vi "Audio.Sound Recorder.vi"() -> ()   [LabVIEW 2018]
uses:
  <vilib>/sound2/lvsound2.llb/Sampling Mode.ctl
  <vilib>/Utility/sysdir.llb/System Directory Type.ctl
  <vilib>/sound2/lvsound2.llb/Sound Input Read (DBL).vi
panel:
  in  "Exit":bool
  out "Active":bool
  in  "Record":bool
  in  "Duration(s)":dbl=5.0 format="%#_13g"
  # "Sound Recorder"
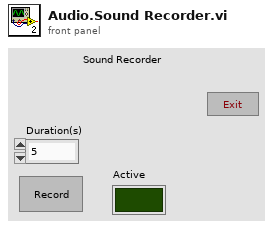
[diagram p1: front panel]
types:
  T1 = typedef "System Directory Type.ctl" = i32
  T2 = typedef "Sampling Mode.ctl" = i32
  T3 = typedef "Sound Input Task ID.ctl" = u32
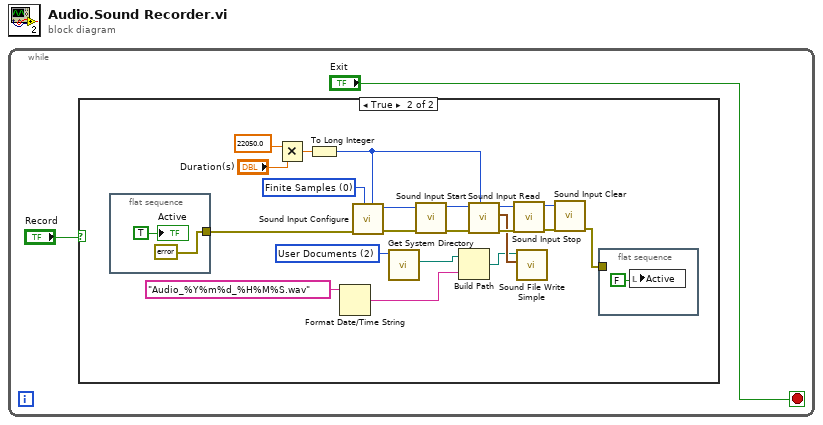
[diagram p0: block diagram]
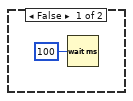
[diagram p2: hidden frame]
diagram:
  n1 = while {
    stop <- "Exit" stop-if-true
    n2 = case shown="True" "Record" {
      frame False {
        n3 = Wait (ms)(milliseconds to wait=u32 100) -> ()  [unwired: 1 out]
      }
      frame True {
        w8 = T1 2 items=["User Home"=0, "User Desktop"=1, "User Documents"=2, "User Application Data"=3, "User Preferences"=4, "User Temporary"=5, "Public Documents"=6, "Public Application Data"=7, "Public Preferences"=8, "Public Cache"=13, "System Core Libraries"=9, "System Installed Libraries"=10, "Application Files"=11, "Boot Volume Root"=12] ("system directory type")
        w22 = T2 0 items=["Finite Samples", "Continuous Samples"] ("sample mode")
        n4 = flat-sequence {
          tunnel: [errorcluster {"status"=FALSE, "code"=0, "source"=""} ("error constant")] -> w4
          frame #0 {
            "Active" <- TRUE ("Active")
          }
        }
        n5 = Multiply(x=22050.0 ("sample rate (S/s)"), y="Duration(s)") -> (x*y=w17:dbl)
        n6 = To Long Integer(number=w17) -> (32bit integer=w16:i32)
        n7 = Format Date/Time String(time format string (%c)="Audio_%Y%m%d_%H%M%S.wav") -> (date/time string=w6:string)  [unwired: 2 in]
        n8 = call <vilib>:"Sound Input Configure.vi"("number of samples/ch"=w16, "sample mode"=w22, "error in (no error)"=w4) -> ("error out"=w23:errorcluster, "task ID"=w24:T3)  [unwired: 7 in]
        n9 = call <vilib>:"Get System Directory.vi"("system directory type"=w8) -> ("system directory"=w9:path)  [unwired: 10 in]
        n10 = call <vilib>:"Sound Input Start.vi"("error in (no error)"=w23, "task ID"=w24) -> ("error out"=w20:errorcluster, "task ID out"=w21:T3)  [unwired: 8 in]
        n11 = Build Path(base path=w9, name or relative path=w6) -> (appended path=w10:path)
        n12 = call-poly <vilib>:"Sound Input Read.vi"("number of samples/ch"=w16, "error in (no error)"=w20, "task ID"=w21) -> ("error out"=w15:errorcluster, "data"=w11:waveform(dbl)[], "task ID out"=w14:T3)  [unwired: 6 in]
        n13 = call <vilib>:"Sound Input Stop.vi"("error in (no error)"=w15, "task ID"=w14) -> ("error out"=w13:errorcluster, "task ID out"=w12:T3)  [unwired: 8 in]
        n14 = call <vilib>:"Sound File Write Simple.vi"("data"=w11, "path"=w10) -> ()  [unwired: 8 in, 2 out]
        n15 = call <vilib>:"Sound Input Clear.vi"("error in (no error)"=w13, "task ID"=w12) -> ("error out"=w5:errorcluster)  [unwired: 9 in]
        n16 = flat-sequence {
          tunnel: w5 -> [_]
          frame #0 {
            n17 = local write "Active"(FALSE ("Active")) -> ()
          }
        }
      }
    }
  }
